vi "doMathThing.vi"(9 "Second number":dbl format="%.2g", 10 "First number":dbl format="%.2g") -> (2 "Result":dbl format="%.2g")   [LabVIEW 2013, in "TestMathLib.lvlib"]
uses:
  TestMathLib.lvlib
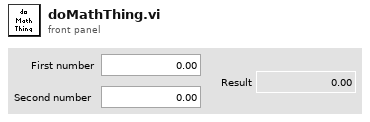
[diagram p1: front panel]
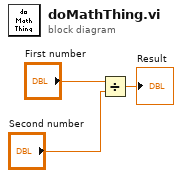
[diagram p0: block diagram]
diagram:
  n1 = Divide(x="First number", y="Second number") -> (x/y=→"Result":dbl)
